vi "GetTrendPoints.vi"(6 "End Time":timestamp, 8 "error in (no error)":errorcluster, 9 "Start Time":timestamp, 10 "trend id":string, 11 "service":refnum<class "IcmMessageService.lvclass">) -> (0 "error out":errorcluster, 3 "TrendPoints":T1[](array[typedef]))   [LabVIEW 2016]
doc: "Queries for the trendpoints in a range for a trend id."
uses:
  <vilib>/addons/InsightCM/MessageBus/MessageService/IcmMessageService.lvclass
  <vilib>/addons/InsightCM/MessageBus/Base/controls/TrendPointQueryParams.ctl
  <vilib>/addons/InsightCM/MessageBus/MessageLibrary/DataManagement/controls/DataManagementQueryTrendPointsRequestBody.ctl
  <vilib>/addons/InsightCM/MessageBus/Base/controls/KeyValuePair.ctl
  <vilib>/addons/InsightCM/MessageBus/Base/controls/TrendPoint.ctl
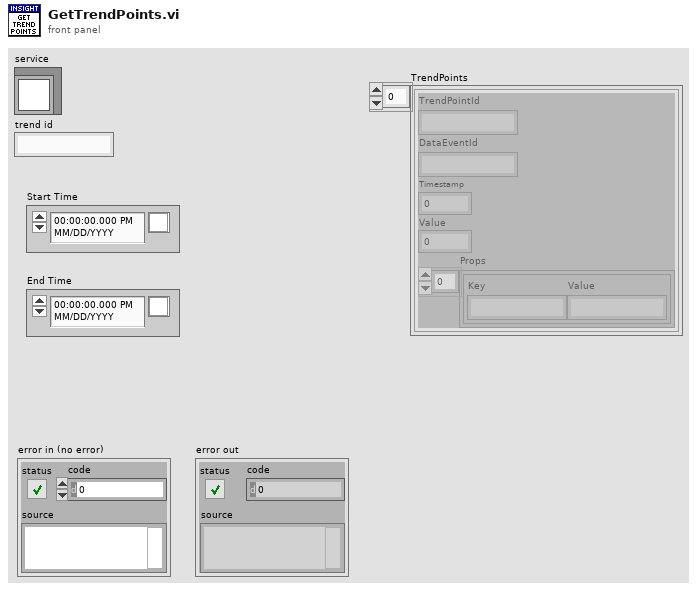
[diagram p1: front panel]
types:
  T1 = typedef "TrendPoint.ctl" = cluster{"TrendPointId":string, "DataEventId":string, "Timestamp":i64, "Value":dbl, "Props":T2[]}
  T2 = typedef "KeyValuePair.ctl" = cluster{"Key":string, "Value":string}
  T3 = typedef "DataManagementQueryTrendPointsRequestBody.ctl" = cluster{"QueryParams":T4}
  T4 = typedef "TrendPointQueryParams.ctl" = cluster{"TrendId":string, "StartTs":i64, "EndTs":i64, "OpState":string}
  T5 = typedef "Message.ctl" = cluster{"Header":T6, "Body":u8[]}
  T6 = typedef "MessageHeader.ctl" = cluster{"MessageName":string, "Timestamp":i64, "CorrelationId":string, "ContentType":string, "RoutingKey":string, "Properties":T2[]}
  T7 = typedef "DataManagementQueryTrendPointsResponseBody.ctl" = cluster{"TrendPoints":T1[]}
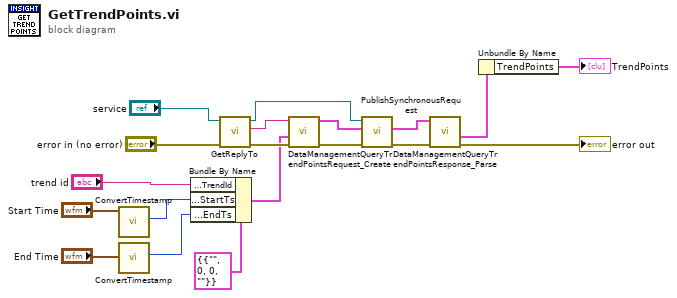
[diagram p0: block diagram]
diagram:
  n1 = call <vilib>:"ConvertTimestamp.vi"("Time Stamp"="Start Time") -> ("Timestamp out"=w3:i64)  [unwired: 10 in]
  n2 = call <vilib>:"ConvertTimestamp.vi"("Time Stamp"="End Time") -> ("Timestamp out"=w2:i64)  [unwired: 10 in]
  n3 = Bundle By Name(cluster=T3 {"QueryParams"={"TrendId"="", "StartTs"=0, "EndTs"=0, "OpState"=""}} ("DataManagementQueryTrendPointsRequest"), "QueryParams.TrendId"="trend id", "QueryParams.StartTs"=w3, "QueryParams.EndTs"=w2) -> (w1:T3)
  n4 = call <vilib>:"GetReplyTo.vi"("error in (no error)"="error in (no error)", "service in"="service") -> ("error out"=w14:errorcluster, "reply to"=w12:string, "service out"=w19:refnum<class "IcmMessageService.lvclass">)  [unwired: 7 in]
  n5 = call <vilib>:"DataManagementQueryTrendPointsRequest_Create.vi"("error in (no error)"=w14, "DataManagementQueryTrendPointsRequest"=w1, "ReplyTo"=w12) -> ("error out"=w13:errorcluster, "Message"=w11:T5)  [unwired: 7 in]
  n6 = call <vilib>:"PublishSynchronousRequest.vi"("error in (no error)"=w13, "request"=w11, "service in"=w19) -> ("error out"=w10:errorcluster, "response"=w7:T5)  [unwired: 6 in, 1 out]
  n7 = call <vilib>:"DataManagementQueryTrendPointsResponse_Parse.vi"("error in (no error)"=w10, "Message"=w7) -> ("error out"=→"error out":errorcluster, "Body"=w8:T7)  [unwired: 6 in, 2 out]
  n8 = Unbundle By Name(w8) -> ("TrendPoints"=→"TrendPoints":T1[])
